vi "ListBox_Facade.vi"(0 "Data In":T6, 2 "Display State In":T2, 3 "Container State":T5) -> (6 "Data Out":T6, 7 "Display State Out":T2, 8 "Action":T1)   [LabVIEW 2012, in "ListBox_XControl.xctl"]
uses:
  ListBox_XControl.xctl
  ListBox_Data.ctl
  <vilib>/_xctls/Container State.ctl
  ListBox_State.ctl
  VIs/Order Type Def.ctl
  VIs/Value Filters.ctl
  <vilib>/_xctls/Action.ctl
  <vilib>/Utility/miscctls.llb/LVRowAndColumnTypeDef.ctl
  <vilib>/_xctls/XControlSupport.lvlib
panel:
  in  "Multicolumn Listbox":i32(listbox)
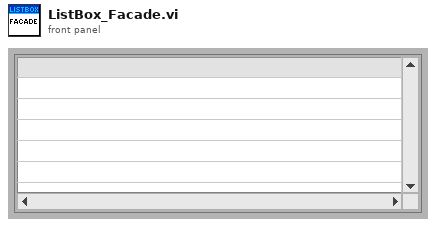
[diagram p1: front panel]
types:
  T1 = typedef "XControlSupport.lvlib/Action.ctl" = cluster{"Data Changed?":bool, "State Changed?":bool, "Action Name":string}
  T2 = typedef "ListBox_XControl.xctl/ListBox_State.ctl" = cluster{"Alternating BG Color":u32, "Alternating Text Color":u32, "Order by Col":i32, "Order":T3, "Value Filters":T4, "Item Names before Filtering":string[][], "Item Names after Filtering":string[][], "Column Header Strings[]":string[], "Column Widths":u32[], "Autosize by Column":i32, "Autosize Activated?":bool, "Autosize Cell Padding":u32}
  T3 = typedef "ListBox_XControl.xctl/Order Type Def.ctl" = enum16{"Ascending", "Descending", "Off"}
  T4 = typedef "ListBox_XControl.xctl/Value Filters.ctl" = cluster{"Column":i32, "Only include Values From":string, "Only include Values to":string}[]
  T5 = typedef "XControlSupport.lvlib/Container State.ctl" = cluster{"Indicator?":bool, "Run Mode?":bool, " Refnum":refnum<vi>}
  T6 = typedef "ListBox_XControl.xctl/ListBox_Data.ctl" = i32
  T7 = typedef "LVRowAndColumnTypeDef.ctl" = cluster{"Row":i32, "Column":i32}
  T8 = typedef "LVFontTypeDef.ctl" = cluster{"Font Name":string, "Size":u16, "Bold":bool, "Italic":bool, "Underline":bool, "Strikeout":bool, "Color":u32}
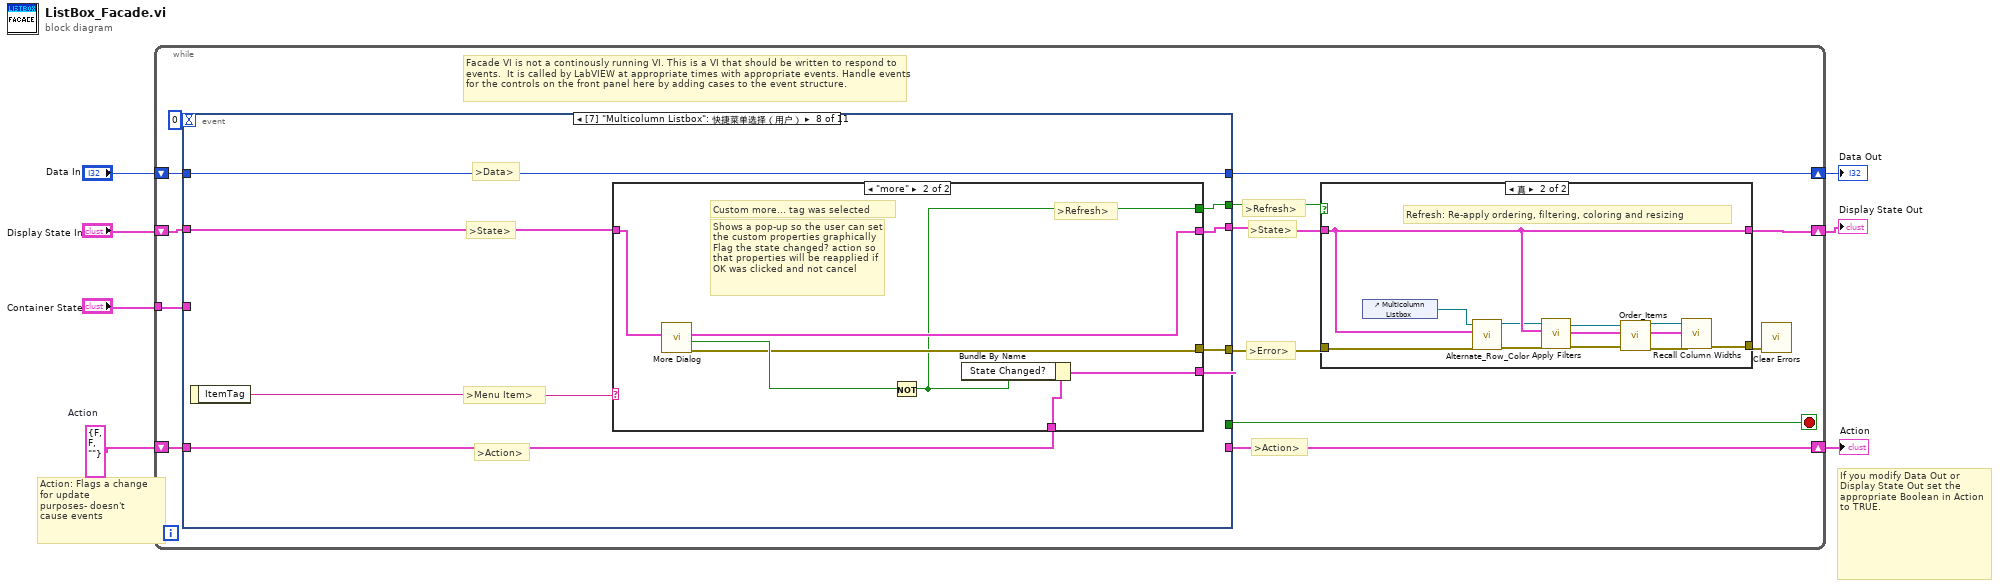
[diagram p0: block diagram]
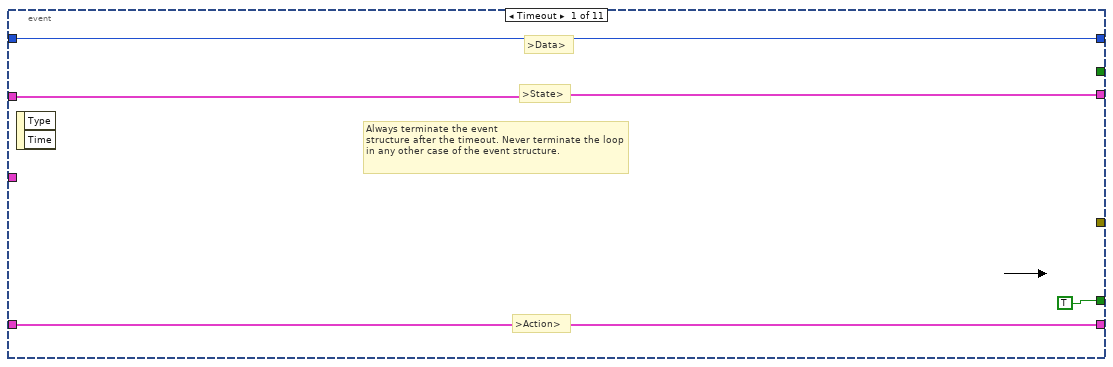
[diagram p3: hidden frame]
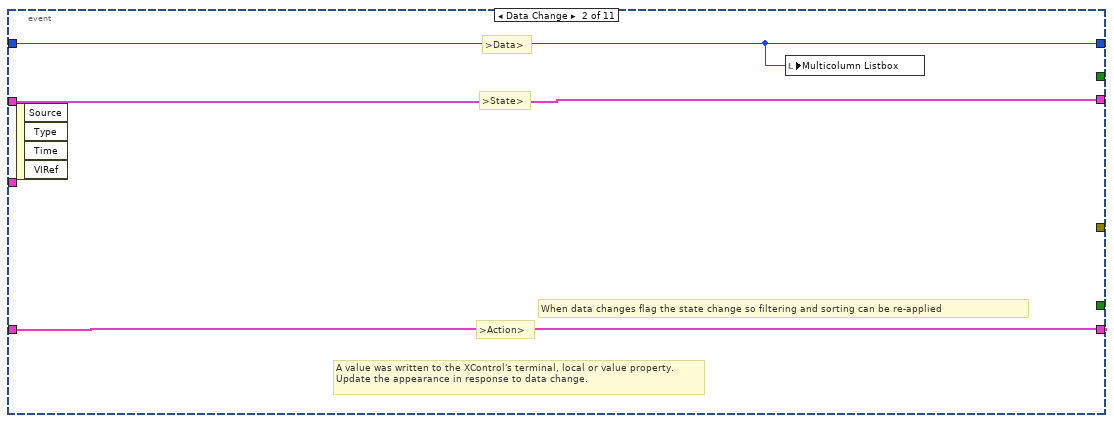
[diagram p4: hidden frame]
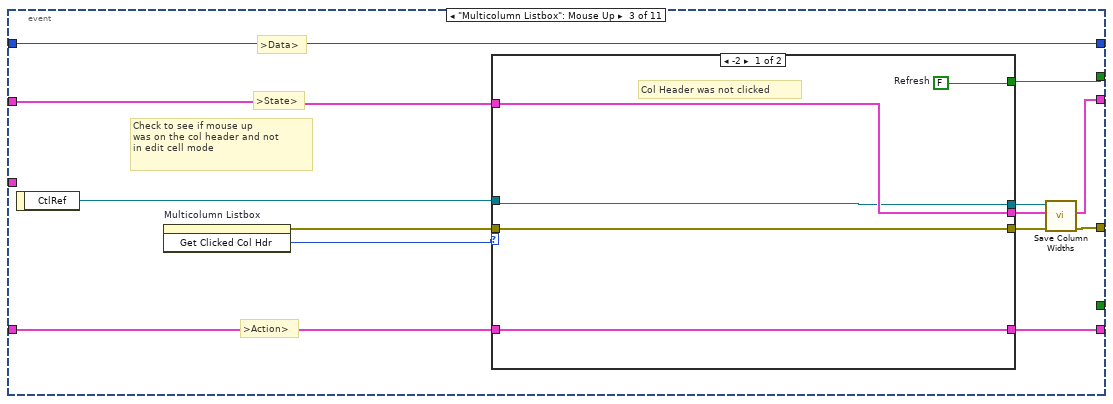
[diagram p5: hidden frame]
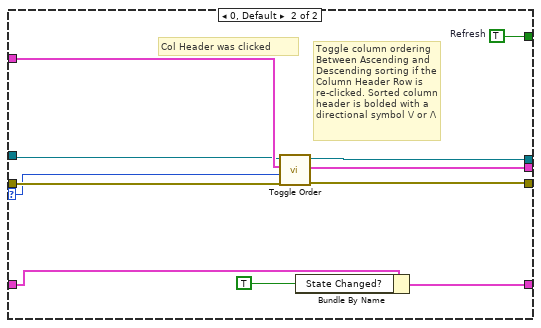
[diagram p6: hidden frame]
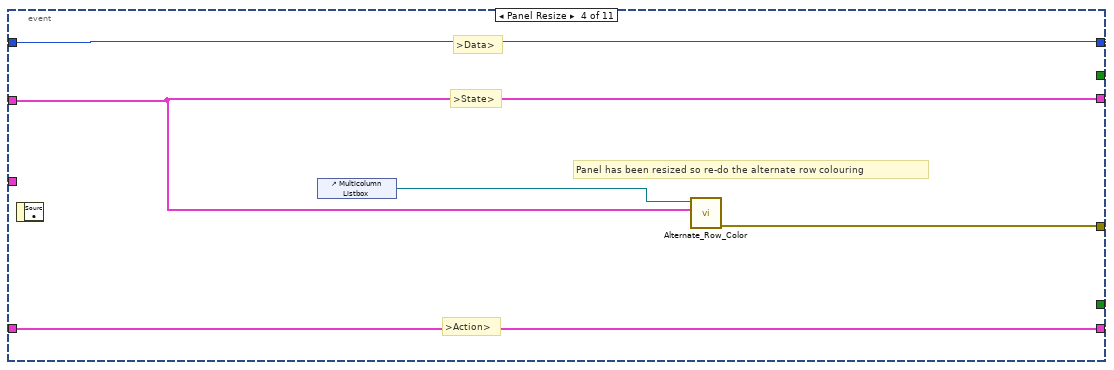
[diagram p7: hidden frame]
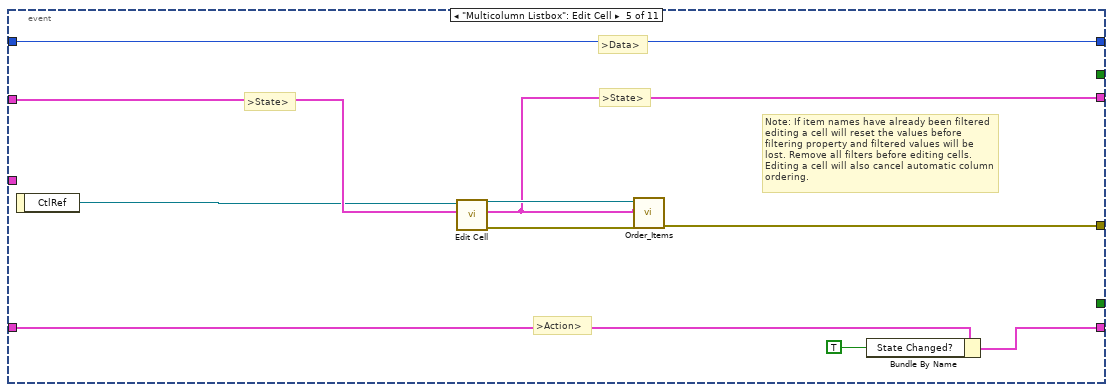
[diagram p8: hidden frame]
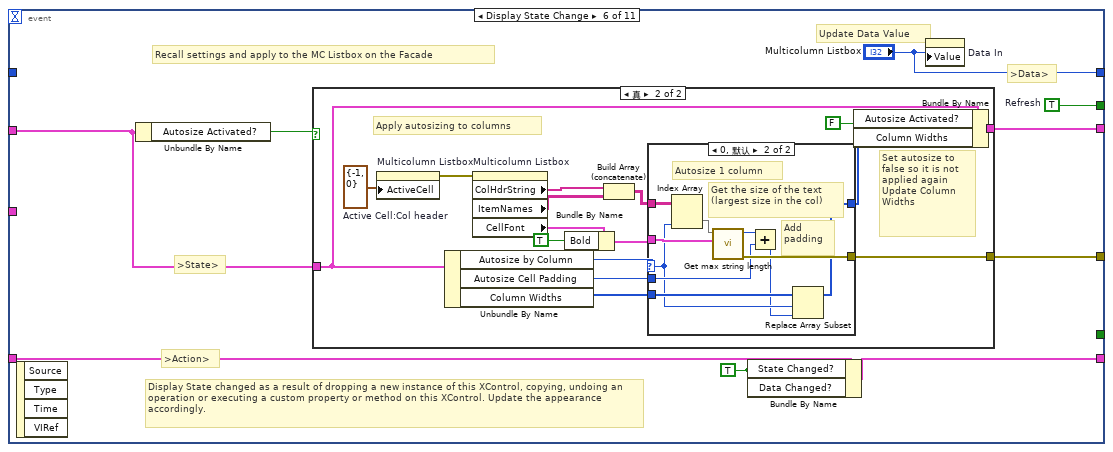
[diagram p9: hidden frame]
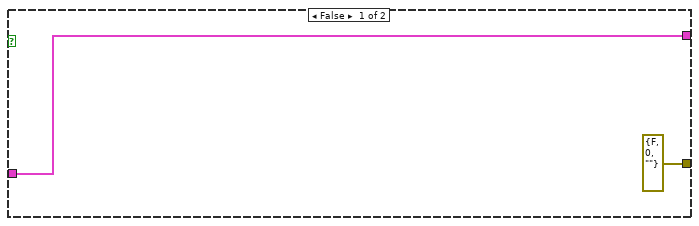
[diagram p10: hidden frame]
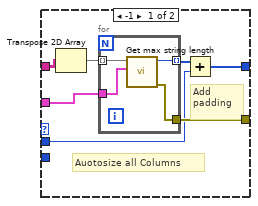
[diagram p11: hidden frame]
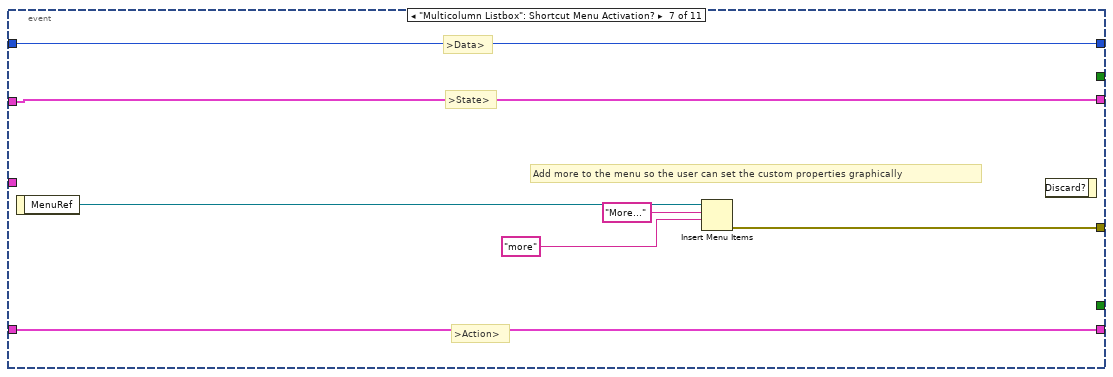
[diagram p12: hidden frame]
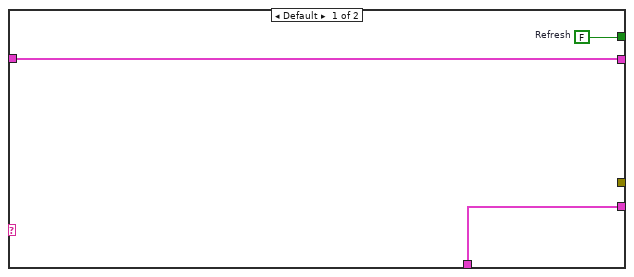
[diagram p13: hidden frame]
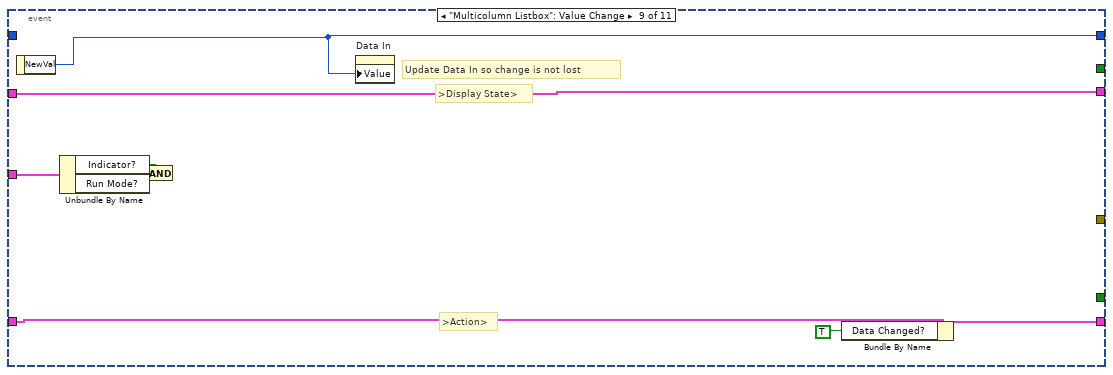
[diagram p14: hidden frame]
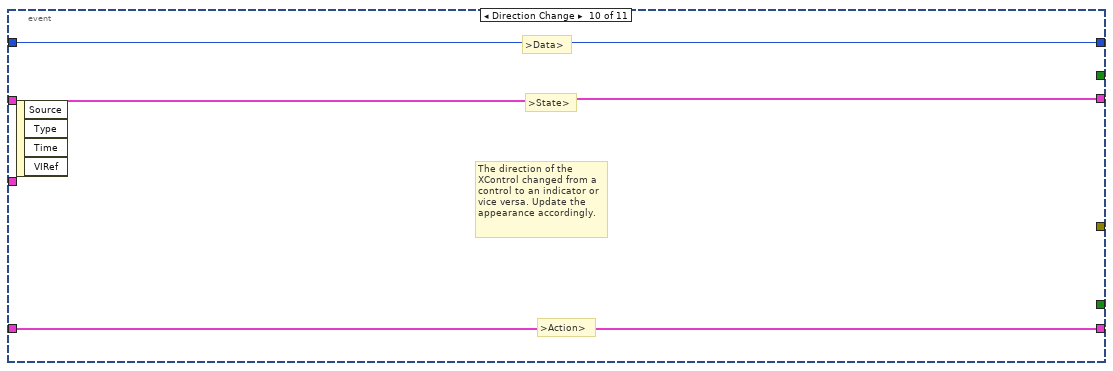
[diagram p15: hidden frame]
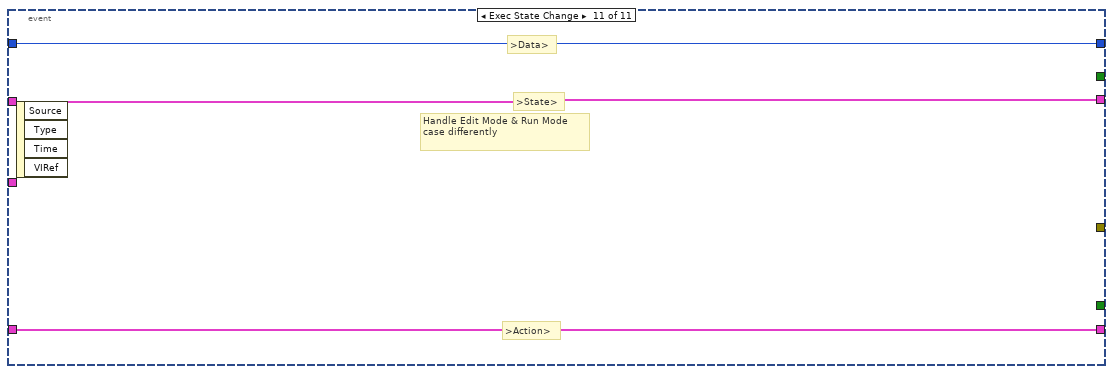
[diagram p16: hidden frame]
diagram:
  w2 = T1 {"Data Changed?"=FALSE, "State Changed?"=FALSE, "Action Name"=""}  # Action
  # "Action: Flags a change\nfor update\npurposes- doesn't\ncause events"
  # "If you modify Data Out or\nDisplay State Out set the\nappropriate Boolean in Action\nto TRUE."
  n1 = while {
    shift-right: [w11] -> w5
    shift-left: "Display State In" -> [w20]
    tunnel: "Container State" -> [w17]
    shift-right: [w15] -> w7
    shift-left: "Data In" -> [w16]
    shift-right: [w13] -> w3
    shift-left: w2 -> [w14]
    stop <- w19 stop-if-true
    # ">Action>"
    # ">State>"
    # ">Error>"
    # ">Refresh>"
    # "Facade VI is not a continously running VI. This is a VI that should be written to respond to events.  It is called by LabVIEW at appropriate times with appropriate events. Handle events for the controls on the front panel here by adding cases to the event structure."
    n2 = event shown="[7] \"Multicolumn Listbox\": 快捷菜单选择（用户）" {
      selector: _ -> [_ _ _ _ _ _ _ _ _ _ _]
      dyn-events: _ -> [_ _ _ _ _ _ _ _ _ _ _]
      timeout: 0 -> [_ _ _ _ _ _ _ _ _ _ _]
      tunnel: w20 -> [w36 w40 w52 w73 w81 w92 w139 w147 w166 w169 w170]
      tunnel: [w36 w40 w47 w73 w78 w90 w139 w144 w166 w169 w170] -> w10
      tunnel: [TRUE _ _ _ _ _ _ _ _ _ _] -> w19
      tunnel: w17 -> [_ _ _ _ _ _ _ _ w165 _ _]
      tunnel: w16 -> [w35 w41 w42 w74 w85 _ w140 w146 _ w168 w172]
      tunnel: [w35 w41 w42 w74 w85 "Multicolumn Listbox" w140 w146 w162 w168 w172] -> w15
      tunnel: [w37 w39 w53 w71 w82 w88 w138 w142 w160 w167 w171] -> w13
      tunnel: w14 -> [w37 w39 w54 w71 w83 w89 w138 w143 w159 w167 w171]
      tunnel: [_ _ w50 w72 w77 w91 w136 w145 _ _ _] -> w12
      tunnel: [_ _ w46 _ _ w94 _ w141 _ _ _] -> w9
      event Timeout {
        # ">Data>"
        # ">State>"
        # ">Action>"
        # "Always terminate the event\nstructure after the timeout. Never terminate the loop in any other case of the event structure."
        n3 = event-data() -> ()  [unwired: 1 in, 2 out]
      }
      event Data Change {
        # ">Action>"
        # ">State>"
        # ">Data>"
        # "When data changes flag the state change so filtering and sorting can be re-applied"
        # "A value was written to the XControl's terminal, local or value property.\nUpdate the appearance in response to data change."
        n4 = event-data() -> ()  [unwired: 1 in, 4 out]
        n5 = local write "Multicolumn Listbox"(w41) -> ()
      }
      event "Multicolumn Listbox": Mouse Up {
        # ">Action>"
        # ">State>"
        # ">Data>"
        # "Check to see if mouse up\nwas on the col header and not\nin edit cell mode"
        n6 = event-data() -> ("CtlRef"=w43:refnum<vi>)  [unwired: 1 in]
        n7 = invoke on="Multicolumn Listbox" class="MCListbox (strict)" method="Get Clicked Col Hdr"() -> (error out=w45:errorcluster, "Get Clicked Column Header"=w44:i32)  [unwired: 3 in, 1 out]
        n8 = case shown="-2" w44 {
          selector: w44 -> [_ w60]
          tunnel: w54 -> [w59 w70]
          tunnel: [w59 w68] -> w53
          tunnel: w52 -> [w58 w67]
          tunnel: [w58 w66] -> w49
          tunnel: w45 -> [w57 w65]
          tunnel: [w57 w63] -> w51
          tunnel: [w55 w62] -> w48
          tunnel: [w56 w64] -> w46
          tunnel: w43 -> [w55 w61]
          frame -2 {
            w56 = FALSE  # Refresh
            # "Col Header was not clicked"
          }
          frame 0, Default {
            w64 = TRUE  # Refresh
            # "Col Header was clicked"
            # "Toggle column ordering Between Ascending and Descending sorting if the Column Header Row is re-clicked. Sorted column header is bolded with a directional symbol \\/ or /\\"
            n9 = call "Toggle Order.vi"("error in (no error)"=w65, "Column"=w60, "Display State In"=w67, "MCListbox Refnum in"=w61) -> ("error out"=w63:errorcluster, "Display State Out"=w66:T2, "MCListbox Refnum  out"=w62:refnum<vi>)  [unwired: 5 in]
            n10 = Bundle By Name(cluster=w70, "State Changed?"=TRUE) -> (w68:T1)
          }
        }
        n11 = call "Save Column Widths.vi"("error in"=w51, "Display State in"=w49, "MCListbox Refnum in"=w48) -> ("error out"=w50:errorcluster, "Display State out"=w47:T2)  [unwired: 5 in, 1 out]
      }
      event Panel Resize {
        # ">Action>"
        # ">State>"
        # ">Data>"
        # "Panel has been resized so re-do the alternate row colouring"
        n12 = event-data() -> ()  [unwired: 1 in, 1 out]
        n13 = control-ref of="Multicolumn Listbox"() -> (w75:refnum<vi>)
        n14 = call "Alternate_Row_Color.vi"("State"=w73, "MCListbox Refnum in"=w75) -> ("error out"=w72:errorcluster)  [unwired: 7 in, 1 out]
      }
      event "Multicolumn Listbox": Edit Cell {
        # ">Action>"
        # ">State>"
        # ">State>"
        # ">Data>"
        # "Note: If item names have already been filtered editing a cell will reset the values before filtering property and filtered values will be lost. Remove all filters before editing cells. Editing a cell will also cancel automatic column ordering."
        n15 = event-data() -> ("CtlRef"=w76:refnum<vi>)  [unwired: 1 in]
        n16 = call "Edit Cell.vi"("Display State In"=w81, "MCListbox Refnum"=w76) -> ("error out"=w80:errorcluster, "Display State out"=w78:T2, "MCListbox Refnum out"=w79:refnum<vi>)  [unwired: 7 in]
        n17 = call "Order_Items.vi"("error in"=w80, "State in"=w78, "MCListbox Refnum in"=w79) -> ("error out"=w77:errorcluster)  [unwired: 5 in, 2 out]
        n18 = Bundle By Name(cluster=w83, "State Changed?"=TRUE) -> (w82:T1)
      }
      event Display State Change {
        w86 = TRUE ("State Changed?")
        w94 = TRUE  # Refresh
        # "Update Data Value"
        # ">Action>"
        # ">State>"
        # ">Data>"
        # "Recall settings and apply to the MC Listbox on the Facade"
        # "Display State changed as a result of dropping a new instance of this XControl, copying, undoing an operation or executing a custom property or method on this XControl. Update the appearance accordingly."
        n19 = event-data() -> ()  [unwired: 1 in, 4 out]
        n20 = Unbundle By Name(w92) -> ("Autosize Activated?"=w93:bool)
        n21 = case shown="真" w93 {
          tunnel: w92 -> [w96 w107]
          tunnel: [errorcluster {"status"=FALSE, "code"=0, "source"=""} ("error out") w111] -> w91
          tunnel: [w96 w108] -> w90
          frame False {
          }
          frame True {
            w100 = T7 {"Row"=-1, "Column"=0}  # Active Cell:Col header
            # "Set autosize to \nfalse so it is not\napplied again\nUpdate Column\nWidths"
            # "Apply autosizing to columns"
            n22 = property on="Multicolumn Listbox" class="MCListbox (严格)"("ActiveCell"=w100) -> (error out=w101:errorcluster)  [unwired: 2 in, 1 out]
            n23 = Unbundle By Name(w107) -> ("Autosize by Column"=w112:i32, "Autosize Cell Padding"=w110:u32, "Column Widths"=w109:u32[])
            n24 = property on="Multicolumn Listbox" class="MCListbox (严格)"(error in=w101) -> ("ColHdrString"=w104:string[], "ItemNames"=w103:string[][], "CellFont"=w99:T8)  [unwired: 1 in, 2 out]
            n25 = Bundle By Name(cluster=w99, "Bold"=TRUE) -> (w98:T8)
            n26 = Build Array (concatenate)(w104, w103) -> (w102:string[][])
            n27 = case shown="0, 默认" w112 {
              selector: w112 -> [_ w126]
              tunnel: w102 -> [w119 w133]
              tunnel: w98 -> [w117 w131]
              tunnel: [w116 w130] -> w111
              tunnel: w110 -> [w114 w128]
              tunnel: w109 -> [_ w127]
              tunnel: [w113 w124] -> w105
              frame -1 {
                # "Add\npadding"
                # "Auotosize all Columns"
                n28 = Transpose 2D Array(2D array=w119) -> (transposed array=w118:string[][])
                n29 = for {
                  tunnel: w118 -> [w123] mode=indexing
                  tunnel: w117 -> [w122]
                  tunnel: [w121] -> w116
                  tunnel: [w120] -> w115 mode=indexing
                  n30 = call "Get max string length.vi"("Font (13pt App)"=w122, "Array of strings"=w123) -> ("error out"=w121:errorcluster, "max width (pixels)"=w120:u32)  [unwired: 8 in]
                }
                n31 = Add(x=w115, y=w114) -> (x+y=w113:u32[])
              }
              frame 0, Default {
                # "Add\npadding"
                # "Autosize 1 column"
                # "Get the size of the text\n(largest size in the col)"
                n32 = Index Array(array=w133, index (col)=w126) -> (element=w132:string[])  [unwired: 1 in]
                n33 = call "Get max string length.vi"("Font (13pt App)"=w131, "Array of strings"=w132) -> ("error out"=w130:errorcluster, "max width (pixels)"=w129:u32)  [unwired: 8 in]
                n34 = Add(x=w129, y=w128) -> (x+y=w125:u32)
                n35 = Replace Array Subset(array=w127, new element=w125, index=w126) -> (w124:u32[])
              }
            }
            n36 = Bundle By Name(cluster=w107, "Autosize Activated?"=FALSE, "Column Widths"=w105) -> (w108:T2)
          }
        }
        n37 = Bundle By Name(cluster=w89, "State Changed?"=w86, "Data Changed?"=w86) -> (w88:T1)
        n38 = property on="Data In" class="DigNum (严格)"("Value"="Multicolumn Listbox") -> ()  [unwired: 2 in, 2 out]
      }
      event "Multicolumn Listbox": Shortcut Menu Activation? {
        # ">Action>"
        # ">State>"
        # ">Data>"
        # "Add more to the menu so the user can set the custom properties graphically"
        n39 = event-data() -> ("MenuRef"=w137:refnum<k9>)  [unwired: 1 in]
        n40 = Insert Menu Items(7:"more", 8:"More...", 9:w137) -> (0:w136:errorcluster)  [unwired: 3 in, 2 out]
        n41 = event-data() -> ()  [unwired: 2 in, 1 out]
      }
      event "Multicolumn Listbox": Shortcut Menu Selection (User) {
        # ">Menu Item>"
        # ">Action>"
        # ">State>"
        # ">Data>"
        n42 = event-data() -> ("ItemTag"=w148:string)  [unwired: 1 in]
        n43 = case shown="\"more\"" w148 {
          tunnel: w147 -> [w151 w156]
          tunnel: [_ w153] -> w145
          tunnel: [w151 w154] -> w144
          tunnel: w143 -> [w150 w158]
          tunnel: [w150 w157] -> w142
          tunnel: [w149 w152] -> w141
          frame Default {
            w149 = FALSE  # Refresh
          }
          frame "more" {
            # ">Refresh>"
            # "Custom more... tag was selected"
            # "Shows a pop-up so the user can set the custom properties graphically\nFlag the state changed? action so that properties will be reapplied if\nOK was clicked and not cancel"
            n44 = call "More Dialog.vi"("State in"=w156) -> ("error out"=w153:errorcluster, "Cancelled?"=w155:bool, "State out"=w154:T2)  [unwired: 8 in]
            n45 = Not(x=w155) -> (.not. x?=w152:bool)
            n46 = Bundle By Name(cluster=w158, "State Changed?"=w152) -> (w157:T1)
          }
        }
      }
      event "Multicolumn Listbox": Value Change {
        # "Update Data In so change is not lost"
        # ">Display State>"
        # ">Action>"
        n47 = event-data() -> ("NewVal"=w162:i32)  [unwired: 1 in]
        n48 = Unbundle By Name(w165) -> ("Indicator?"=w164:bool, "Run Mode?"=w163:bool)
        n49 = And(x=w164, y=w163) -> ()  [unwired: 1 out]
        n50 = property on="Data In" class="DigNum (严格)"("Value"=w162) -> ()  [unwired: 2 in, 2 out]
        n51 = Bundle By Name(cluster=w159, "Data Changed?"=TRUE) -> (w160:T1)
      }
      event Direction Change {
        # ">Action>"
        # ">State>"
        # ">Data>"
        # "The direction of the XControl changed from a control to an indicator or vice versa. Update the appearance accordingly."
        n52 = event-data() -> ()  [unwired: 1 in, 4 out]
      }
      event Exec State Change {
        # ">Action>"
        # ">State>"
        # ">Data>"
        # "Handle Edit Mode & Run Mode\ncase differently"
        n53 = event-data() -> ()  [unwired: 1 in, 4 out]
      }
    }
    n54 = case shown="真" w9 {
      tunnel: w12 -> [w21 w33]
      tunnel: [w22 w24] -> w11
      tunnel: w10 -> [w22 w24]
      tunnel: [w21 w32] -> w8
      frame False {
      }
      frame True {
        # "Refresh: Re-apply ordering, filtering, coloring and resizing"
        n55 = control-ref of="Multicolumn Listbox"() -> (w34:refnum<vi>)
        n56 = call "Alternate_Row_Color.vi"("error in"=w33, "State"=w24, "MCListbox Refnum in"=w34) -> ("error out"=w31:errorcluster, "MCListbox Refnum out"=w23:refnum<vi>)  [unwired: 6 in]
        n57 = call "Apply Filters.vi"("error in"=w31, "Display State In"=w24, "MCListbox Refnum in"=w23) -> ("error out"=w30:errorcluster, "Display State out"=w25:T2, "MCListbox Refnum out"=w26:refnum<vi>)  [unwired: 6 in]
        n58 = call "Order_Items.vi"("error in"=w30, "State in"=w25, "MCListbox Refnum in"=w26) -> ("error out"=w29:errorcluster, "State out"=w28:T2, "MCListbox Refnum out"=w27:refnum<vi>)  [unwired: 5 in]
        n59 = call "Recall Column Widths.vi"("error in"=w29, "Display State in"=w28, "MCListbox Refnum in"=w27) -> ("error out"=w32:errorcluster)  [unwired: 6 in, 1 out]
      }
    }
    n60 = call <vilib>:"Clear Errors.vi"("error in (no error)"=w8) -> ()  [unwired: 6 in, 1 out]
  }
  "Display State Out" <- w5
  "Data Out" <- w7
  "Action" <- w3
